vi "Data Buffer Test Program.vi"   [LabVIEW 2022 SP3]
uses:
  Data Buffer.lvclass
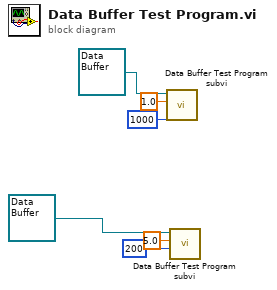
[diagram p0: block diagram]
diagram:
  n1 = call "Data Buffer Test Program subvi.vi"("millisecond multiple"=u32 1000, "Mult"=1.0, "Data Buffer in"=refnum<class "Data Buffer.lvclass"> refnum) -> ()  [unwired: 9 in]
  n2 = call "Data Buffer Test Program subvi.vi"("millisecond multiple"=u32 200, "Mult"=5.0, "Data Buffer in"=refnum<class "Data Buffer.lvclass"> refnum) -> ()  [unwired: 9 in]
